vi "Device to Color.vi"(1 "Device #":string) -> (0 "Color":u32)   [LabVIEW 2020]
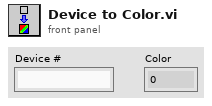
[diagram p1: front panel]
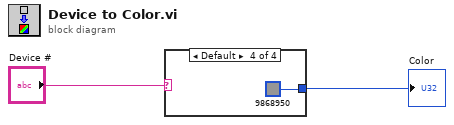
[diagram p0: block diagram]
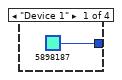
[diagram p2: hidden frame]
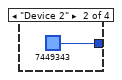
[diagram p3: hidden frame]
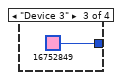
[diagram p4: hidden frame]
diagram:
  n1 = case shown="Default" "Device #" {
    tunnel: [u32 5898187 u32 7449343 u32 16752849 u32 9868950] -> w2
    frame "Device 1" {
    }
    frame "Device 2" {
    }
    frame "Device 3" {
    }
    frame Default {
    }
  }
  "Color" <- w2
